vi "All Keyed Array VIs.vi"() -> ()   [LabVIEW 2011]
panel:
  out "KA XML Children":string
  out "KA String":string
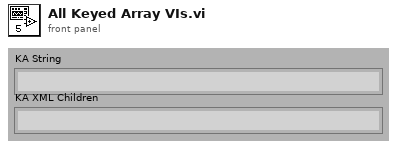
[diagram p1: front panel]
types:
  T1 = typedef "Tools_KeyedArray KeyedArray.ctl" = cluster{"keys":string[], "values":string[]}
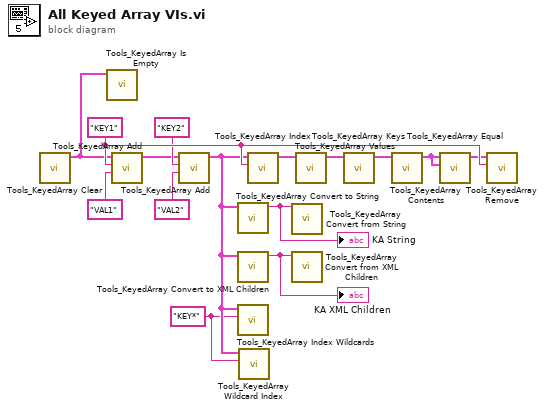
[diagram p0: block diagram]
diagram:
  w2 = "KEY*" ("key")
  w11 = "KEY1" ("key")
  n1 = call "Tools_KeyedArray Clear.vi"() -> ("array out"=w1:T1)  [unwired: 1 in, 6 out]
  n2 = call "Tools_KeyedArray Is Empty.vi"("array in"=w1) -> ()  [unwired: 7 out]
  n3 = call "Tools_KeyedArray Add.vi"("value"="VAL1" ("key"), "key"=w11, "array in"=w1) -> ("array out"=w4:T1)  [unwired: 1 in, 3 out]
  n4 = call "Tools_KeyedArray Add.vi"("value"="VAL2" ("key"), "key"="KEY2", "array in"=w4) -> ("array out"=w3:T1)  [unwired: 1 in, 3 out]
  n5 = call "Tools_KeyedArray Convert to String.vi"("Keyed Array"=w3) -> ("KA String"=w8:string)  [unwired: 10 out]
  "KA String" <- w8
  n6 = call "Tools_KeyedArray Convert to XML Children.vi"("Keyed Array"=w3) -> ("KA XML Children"=w7:string)  [unwired: 10 out]
  "KA XML Children" <- w7
  n7 = call "Tools_KeyedArray Index Wildcards.vi"("key"=w2, "array in"=w3) -> ()  [unwired: 2 in, 4 out]
  n8 = call "Tools_KeyedArray Wildcard Index.vi"("wildcard key"=w2, "array in"=w3) -> ()  [unwired: 2 in, 4 out]
  n9 = call "Tools_KeyedArray Index.vi"("key"=w11, "array in"=w3) -> ("duplicate array"=w15:T1)  [unwired: 2 in, 3 out]
  n10 = call "Tools_KeyedArray Convert from String.vi"("KA String"=w8) -> ()  [unwired: 1 in, 10 out]
  n11 = call "Tools_KeyedArray Convert from XML Children.vi"("KA String"=w7) -> ()  [unwired: 1 in, 10 out]
  n12 = call "Tools_KeyedArray Values.vi"("array in"=w15) -> ("duplicate array"=w14:T1)  [unwired: 6 out]
  n13 = call "Tools_KeyedArray Keys.vi"("array in"=w14) -> ("duplicate array"=w13:T1)  [unwired: 6 out]
  n14 = call "Tools_KeyedArray Contents.vi"("array in"=w13) -> ("duplicate array"=w9:T1)  [unwired: 6 out]
  n15 = call "Tools_KeyedArray Equal.vi"("array B"=w9, "array A"=w9) -> ("duplicate array A"=w10:T1)  [unwired: 2 in, 3 out]
  n16 = call "Tools_KeyedArray Remove.vi"("key"=w11, "array in"=w10) -> ()  [unwired: 1 in, 5 out]
